vi "GDSString_FindCodeBlock.vi"(0 "Text":string, 1 "StringStartOffset(Default=-1 => 0 for Forward, StrLenght for Backwards)":i32=-1, 2 "CodeBlockStartCharacter( { )":string="{", 3 "CodeBlockEndCharacter( } )":string="}", 4 "Search Backwards":bool, 5 "error in (no error)":errorcluster, 7 "SkipBlockCharactersInsideCommentBlocks/*...*/ and //... (True)":bool=TRUE) -> (10 "TextBeforeBlock":string, 11 "TextAfterBlock":string, 13 "found":bool, 14 "BlockText":string, 15 "BlockStart(Outside)":i32, 16 "BlockStart(Inside)":i32, 17 "BlockEnd(Inside)":i32, 18 "BlockEnd(Outside)":i32, 19 "error out":errorcluster)   [LabVIEW 2012]
uses:
  <vilib>/regexp/Match Regular Expression.xnode
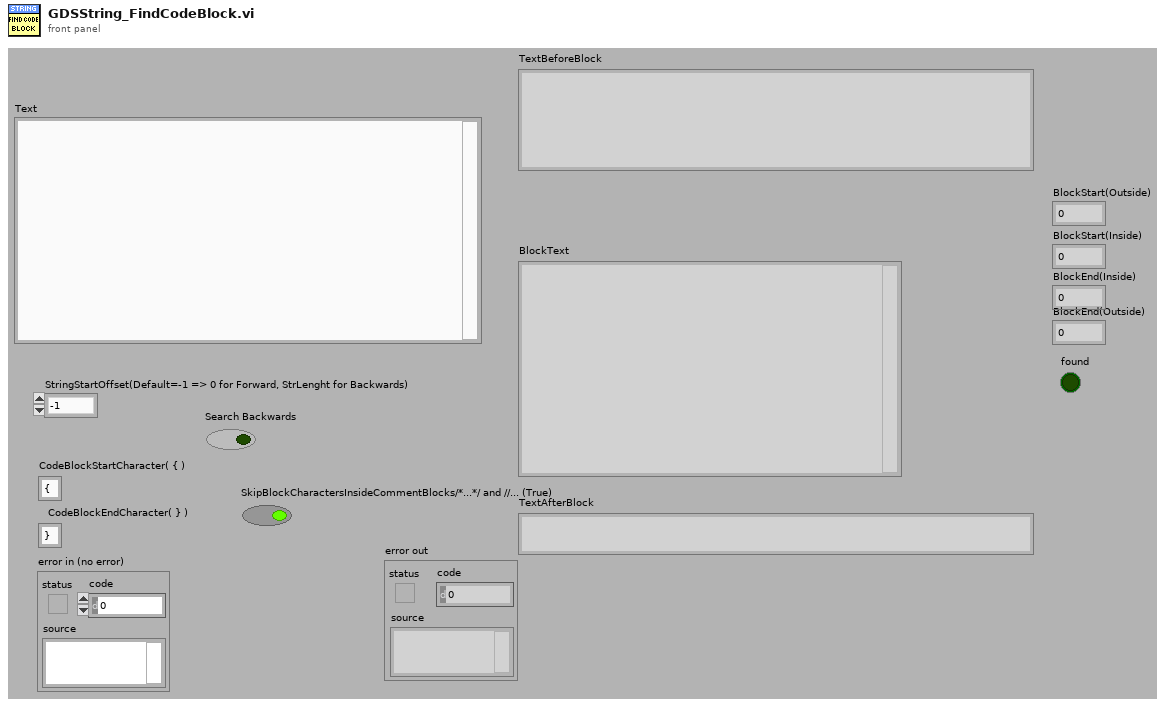
[diagram p1: front panel]
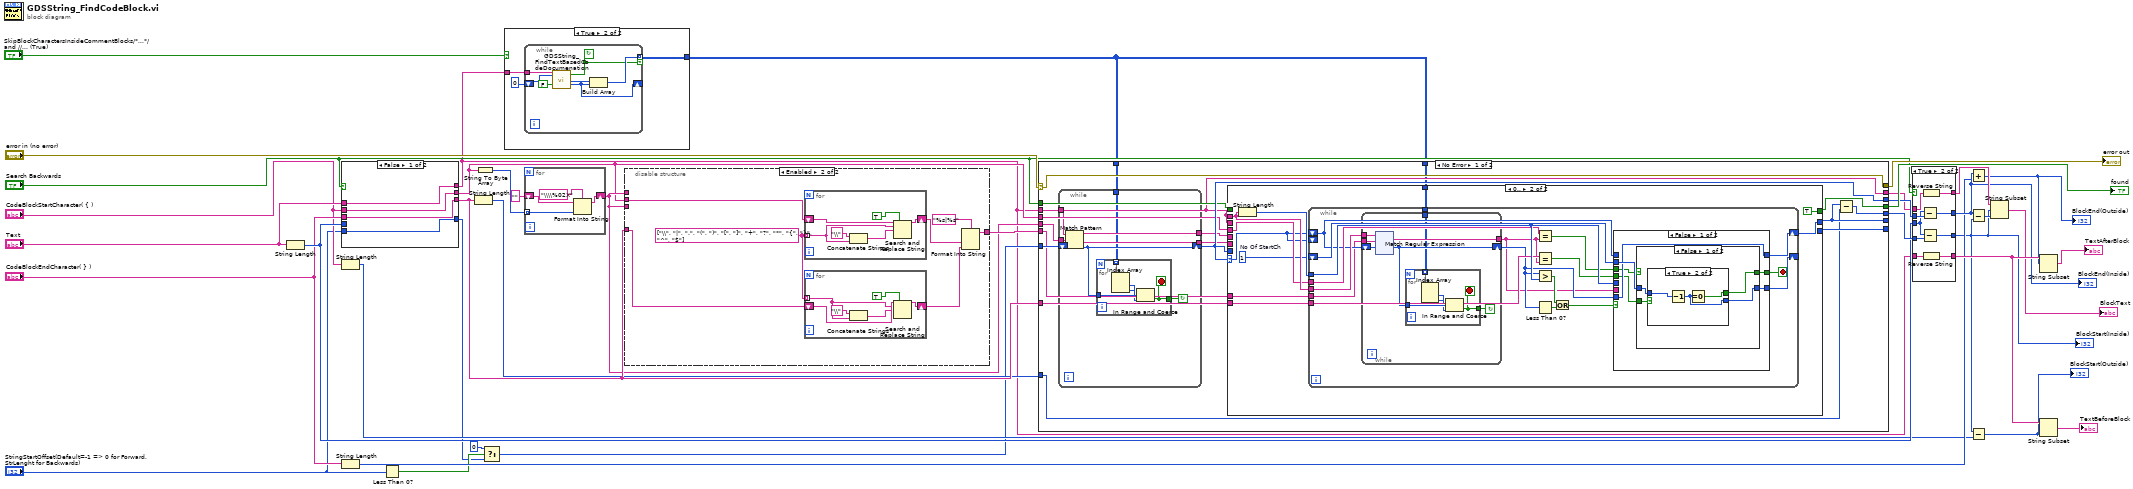
[diagram p0: block diagram]
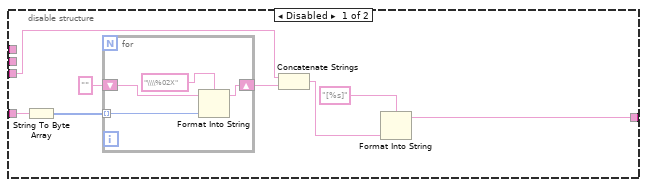
[diagram p3: hidden frame]
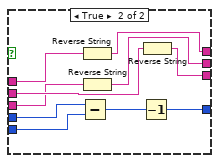
[diagram p5: hidden frame]
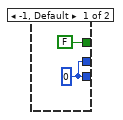
[diagram p6: hidden frame]
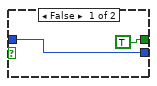
[diagram p7: hidden frame]
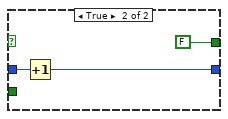
[diagram p8: hidden frame]
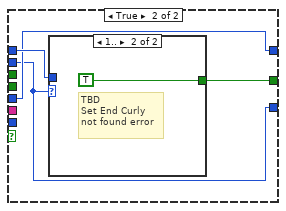
[diagram p9: hidden frame]
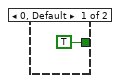
[diagram p10: hidden frame]
diagram:
  n1 = String Length(string="Text") -> (length=w27:i32)
  n2 = case shown="False" "Search Backwards" {
    tunnel: "Text" -> [w42 w47]
    tunnel: [w42 w50] -> w3
    tunnel: "CodeBlockStartCharacter( { )" -> [w41 w52]
    tunnel: [w41 w48] -> w9
    tunnel: "StringStartOffset(Default=-1 => 0 for Forward, StrLenght for Backwards)" -> [w40 w46]
    tunnel: [w40 w44] -> w5
    tunnel: "CodeBlockEndCharacter( } )" -> [w39 w51]
    tunnel: [w39 w49] -> w23
    tunnel: w27 -> [_ w43]
    frame False {
    }
    frame True {
      n3 = Subtract(x=w43, y=w46) -> (x-y=w45:i32)
      n4 = Reverse String(1:w47) -> (0:w50:string)
      n5 = Reverse String(1:w51) -> (0:w48:string)
      n6 = Decrement(x=w45) -> (x-1=w44:i32)
      n7 = Reverse String(1:w52) -> (0:w49:string)
    }
  }
  n8 = String Length(string="CodeBlockStartCharacter( { )") -> (length=w13:i32)
  n9 = String Length(string="CodeBlockEndCharacter( } )") -> (length=w15:i32)
  n10 = Less Than 0?(x="StringStartOffset(Default=-1 => 0 for Forward, StrLenght for Backwards)") -> (x < 0?=w7:bool)
  n11 = String Length(string=w23) -> (length=w22:i32)
  n12 = String To Byte Array(string=w9) -> (unsigned byte array=w35:u8[])
  n13 = Select(t=0, s=w7, f=w5) -> (s? t:f=w6:i32)
  n14 = case shown="True" "SkipBlockCharactersInsideCommentBlocks/*...*/ and //... (True)" {
    tunnel: w3 -> [_ w54]
    tunnel: [_ w53] -> w1
    frame False {
    }
    frame True {
      n15 = while {
        tunnel: w54 -> [w62]
        shift-right: [w60] -> _
        shift-left: 0 ("offset past match") -> [w59]
        tunnel: [w58] -> w53 mode=indexing if=w57
        stop <- w57 continue-if-true
        n16 = call <resource>:"GDSString_FindTextBasedCodeDocumenation.vi"("Text"=w62, "StringStartOffset(Default=-1 => 0 for Forward, StrLenght for Backwards)"=w59, "CommentHasToBeTheFirstItem(True)"=FALSE) -> ("Found"=w57:bool, "IndexBeforeDocument(Or after when searching Backwards)"=w61:i32, "IndexAfterDocument(Or before when searching Backwards)"=w60:i32)  [unwired: 12 in, 2 out]
        n17 = Build Array(w61, w60) -> (w58:i32[])
      }
    }
  }
  n18 = for {
    tunnel: w35 -> [w65] mode=indexing
    shift-right: [w64] -> w11
    shift-left: "" -> [w63]
    n19 = Format Into String(format string="\\\\%02X", initial string=w63, w65) -> (resulting string=w64:string)  [unwired: 1 in, 1 out]
  }
  n20 = disable-structure shown="Enabled" {
    disable-tunnel: w11 -> [w72 _]
    disable-tunnel: [w69 w80] -> w33
    disable-tunnel: w23 -> [w67 w82]
    disable-tunnel: w11 -> [_ _]
    disable-tunnel: w9 -> [_ w79]
    frame Disabled {
      n21 = String To Byte Array(string=w67) -> (unsigned byte array=w73:u8[])
      n22 = for {
        tunnel: w73 -> [w77] mode=indexing
        shift-right: [w76] -> w71
        shift-left: "" -> [w75]
        n23 = Format Into String(format string="\\\\%02X", initial string=w75, w77) -> (resulting string=w76:string)  [unwired: 1 in, 1 out]
      }
      n24 = Concatenate Strings(w72, w71) -> (w70:string)
      n25 = Format Into String(format string="[%s]", w70) -> (resulting string=w69:string)  [unwired: 2 in, 1 out]
    }
    frame Enabled {
      w83 = string[] ["\\", "|", ".", "(", ")", "[", "]", "+", "?", "*", "{", "}", "^", "$"] ("Array")
      n26 = for {
        shift-right: [w95] -> w84
        shift-left: w79 -> [w96]
        tunnel: w83 -> [w94] mode=indexing
        n27 = Concatenate Strings("\\" ("string"), w94) -> (w92:string)
        n28 = Search and Replace String(replace all?=TRUE ("replace all? (F)"), input string=w96, search string=w94, replace string=w92) -> (result string=w95:string)  [unwired: 4 in, 3 out]
      }
      n29 = for {
        shift-right: [w89] -> w81
        shift-left: w82 -> [w90]
        tunnel: w83 -> [w88] mode=indexing
        n30 = Concatenate Strings("\\" ("string"), w88) -> (w86:string)
        n31 = Search and Replace String(replace all?=TRUE ("replace all? (F)"), input string=w90, search string=w88, replace string=w86) -> (result string=w89:string)  [unwired: 4 in, 3 out]
      }
      n32 = Format Into String(format string="%s|%s", w84, w81) -> (resulting string=w80:string)  [unwired: 2 in, 1 out]
    }
  }
  n33 = case shown="No Error" "error in (no error)" {
    selector: "error in (no error)" -> [w109 w306]
    tunnel: [w115 _] -> _
    tunnel: [w114 _] -> w38
    tunnel: w3 -> [w100 _]
    tunnel: [w113 _] -> _
    tunnel: [w100 _] -> w31
    tunnel: [w112 _] -> w30
    tunnel: [w111 _] -> w32
    tunnel: w6 -> [w110 _]
    tunnel: [w109 w306] -> w36
    tunnel: w11 -> [w108 _]
    tunnel: w33 -> [w107 _]
    tunnel: w9 -> [w106 _]
    tunnel: w23 -> [w105 _]
    tunnel: "Search Backwards" -> [w104 _]
    tunnel: w22 -> [w101 _]
    tunnel: w1 -> [w99 _]
    tunnel: w1 -> [w98 _]
    frame No Error {
      n34 = while {
        tunnel: w108 -> [w122]
        tunnel: [w121] -> w103
        tunnel: [w120] -> w102
        tunnel: w100 -> [w119]
        shift-right: [w118] -> w111
        shift-left: w110 -> [w123]
        tunnel: w98 -> [w117]
        stop <- w116 continue-if-true
        n35 = Match Pattern(string=w119, regular expression=w122, offset (0)=w123) -> (before substring=w121:string, after substring=w120:string, offset past match=w118:i32)  [unwired: 1 out]
        n36 = for {
          tunnel: w117 -> [w127] mode=indexing
          tunnel: w118 -> [w128]
          tunnel: [w124] -> w116
          stop <- w124 stop-if-true
          n37 = Index Array(array=w127) -> (element #1=w126:i32, element #2=w125:i32)  [unwired: 2 in]
          n38 = In Range and Coerce(upper limit=w125, x=w128, lower limit=w126) -> (In Range?=w124:bool)  [unwired: 1 out]
        }
      }
      n39 = case shown="0.." w111 {
        selector: w111 -> [_ w132]
        tunnel: w100 -> [_ w140]
        tunnel: [FALSE TRUE] -> w114
        tunnel: w103 -> [_ _]
        tunnel: w111 -> [_ _]
        tunnel: [w129 w133] -> w113
        tunnel: [w129 _] -> w115
        tunnel: w107 -> [_ w137]
        tunnel: w106 -> [_ w136]
        tunnel: w105 -> [_ w135]
        tunnel: w102 -> [_ _]
        tunnel: w104 -> [_ _]
        tunnel: w100 -> [_ _]
        tunnel: w99 -> [_ w131]
        frame -1, Default {
          w129 = 0
        }
        frame 0.. {
          w134 = 1  # No Of StartCh
          n40 = String Length(string=w140) -> (length=w139:i32)
          n41 = while {
            shift-left: w132 -> [_]
            tunnel: w139 -> [w155]
            tunnel: w137 -> [w144]
            tunnel: w140 -> [w146]
            shift-left: w132 -> [w145]
            shift-right: [w154] -> w133
            shift-left: w134 -> [w158]
            shift-right: [w157] -> _
            tunnel: w136 -> [w150]
            tunnel: w135 -> [w147]
            tunnel: w131 -> [w141]
            stop <- w156 stop-if-true
            n42 = while {
              tunnel: w146 -> [w165]
              shift-right: [w161] -> w143
              shift-left: w145 -> [w164]
              tunnel: w144 -> [w163]
              tunnel: [w162] -> w142
              tunnel: w141 -> [w160]
              stop <- w159 continue-if-true
              n43 = xnode "Match Regular Expression"("input string"=w165, "regular expression"=w163, "offset (0)"=w164) -> ("whole match"=w162:string, "offset past match"=w161:i32)  [unwired: 3 in, 3 out]
              n44 = for {
                tunnel: w160 -> [w169] mode=indexing
                tunnel: w161 -> [w170]
                tunnel: [w166] -> w159
                stop <- w166 stop-if-true
                n45 = Index Array(array=w169) -> (element #1=w168:i32, element #2=w167:i32)  [unwired: 2 in]
                n46 = In Range and Coerce(upper limit=w167, x=w170, lower limit=w168) -> (In Range?=w166:bool)  [unwired: 1 out]
              }
            }
            n47 = Equal?(x=w150, y=w142) -> (x = y?=w149:bool)
            n48 = Equal?(x=w147, y=w142) -> (x = y?=w148:bool)
            n49 = Greater?(x=w143, y=w155) -> (0:w153:bool)
            n50 = Less Than 0?(x=w143) -> (x < 0?=w151:bool)
            n51 = Or(x=w153, y=w151) -> (x .or. y?=w152:bool)
            n52 = case shown="False" w152 {
              tunnel: w158 -> [w287 w300]
              tunnel: w145 -> [_ w303]
              tunnel: w142 -> [_ _]
              tunnel: [w286 w300] -> w157
              tunnel: [w285 w301] -> w156
              tunnel: w143 -> [w284 _]
              tunnel: w155 -> [_ w302]
              tunnel: [w284 w302] -> w154
              tunnel: w149 -> [w283 _]
              tunnel: w148 -> [w282 _]
              frame False {
                n53 = case shown="False" w283 {
                  tunnel: w287 -> [w291 w299]
                  tunnel: [w290 w298] -> w286
                  tunnel: [w289 FALSE] -> w285
                  tunnel: w282 -> [w288 _]
                  frame False {
                    n54 = case shown="True" w288 {
                      tunnel: w291 -> [w293 w296]
                      tunnel: [w293 w295] -> w290
                      tunnel: [TRUE w294] -> w289
                      frame False {
                      }
                      frame True {
                        n55 = Decrement(x=w296) -> (x-1=w295:i32)
                        n56 = Equal To 0?(x=w295) -> (x = 0?=w294:bool)
                      }
                    }
                  }
                  frame True {
                    n57 = Increment(x=w299) -> (x+1=w298:i32)
                  }
                }
              }
              frame True {
                n58 = case shown="1.." w300 {
                  tunnel: w303 -> [_ _]
                  tunnel: [TRUE TRUE] -> w301
                  frame 0, Default {
                  }
                  frame 1.. {
                    # "TBD\nSet End Curly\nnot found error"
                  }
                }
              }
            }
          }
        }
      }
      n59 = Subtract(x=w113, y=w101) -> (x-y=w112:i32)
    }
    frame Error {
    }
  }
  "found" <- w38
  "error out" <- w36
  n60 = case shown="True" "Search Backwards" {
    tunnel: w3 -> [w310 w319]
    tunnel: w32 -> [w309 w316]
    tunnel: w31 -> [w308 w318]
    tunnel: w30 -> [w307 w315]
    tunnel: [w310 w313] -> w24
    tunnel: [w309 w311] -> w14
    tunnel: [w308 w317] -> w21
    tunnel: [w307 w312] -> w18
    tunnel: w27 -> [_ w314]
    frame False {
    }
    frame True {
      n61 = Subtract(x=w314, y=w316) -> (x-y=w312:i32)
      n62 = Subtract(x=w314, y=w315) -> (x-y=w311:i32)
      n63 = Reverse String(1:w318) -> (0:w317:string)
      n64 = Reverse String(1:w319) -> (0:w313:string)
    }
  }
  "BlockStart(Inside)" <- w14
  "BlockEnd(Inside)" <- w18
  n65 = Add(x=w18, y=w15) -> (x+y=w10:i32)
  "BlockEnd(Outside)" <- w10
  n66 = Subtract(x=w18, y=w14) -> (x-y=w19:i32)
  n67 = Subtract(x=w14, y=w13) -> (x-y=w12:i32)
  "BlockStart(Outside)" <- w12
  n68 = String Subset(string=w21, offset (0)=w14, length (rest)=w19) -> (substring=→"BlockText":string)
  n69 = String Subset(string=w24, offset (0)=w10) -> (substring=→"TextAfterBlock":string)  [unwired: 1 in]
  n70 = String Subset(string=w24, length (rest)=w12) -> (substring=→"TextBeforeBlock":string)  [unwired: 1 in]
